vi "sub_qam_symbol_map_gen.vi"(9 "Gray code?":bool, 11 "M-QAM":i32) -> (3 "symbol map":cdb[](array[numeric]))   [LabVIEW 2014]
panel:
  out "Gray coded map":u32[][](array[numeric])
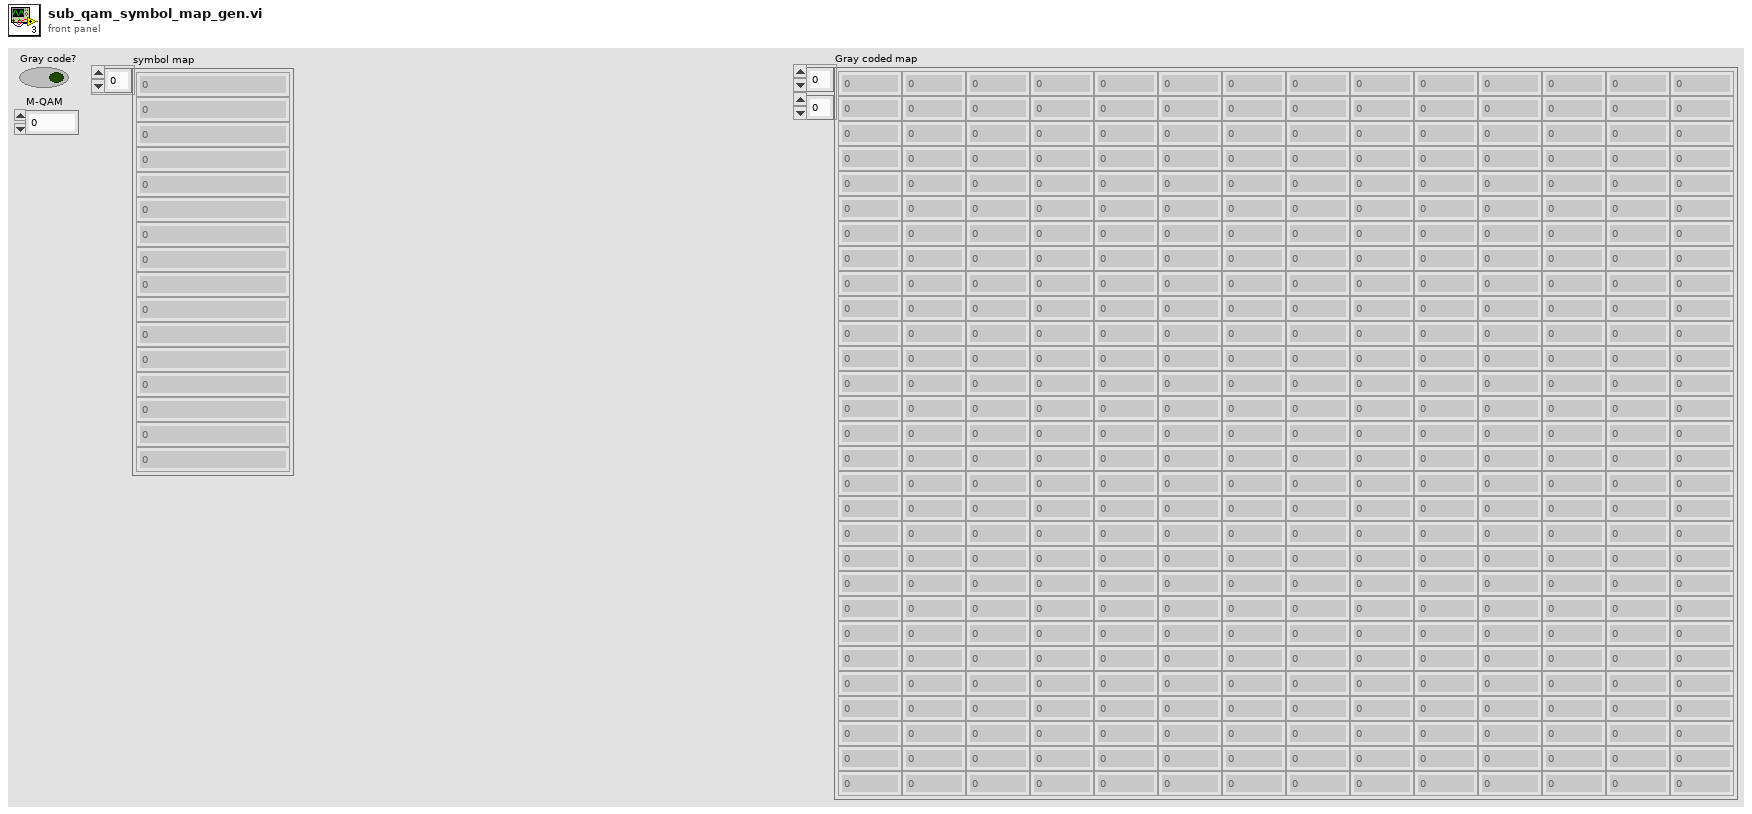
[diagram p1: front panel]
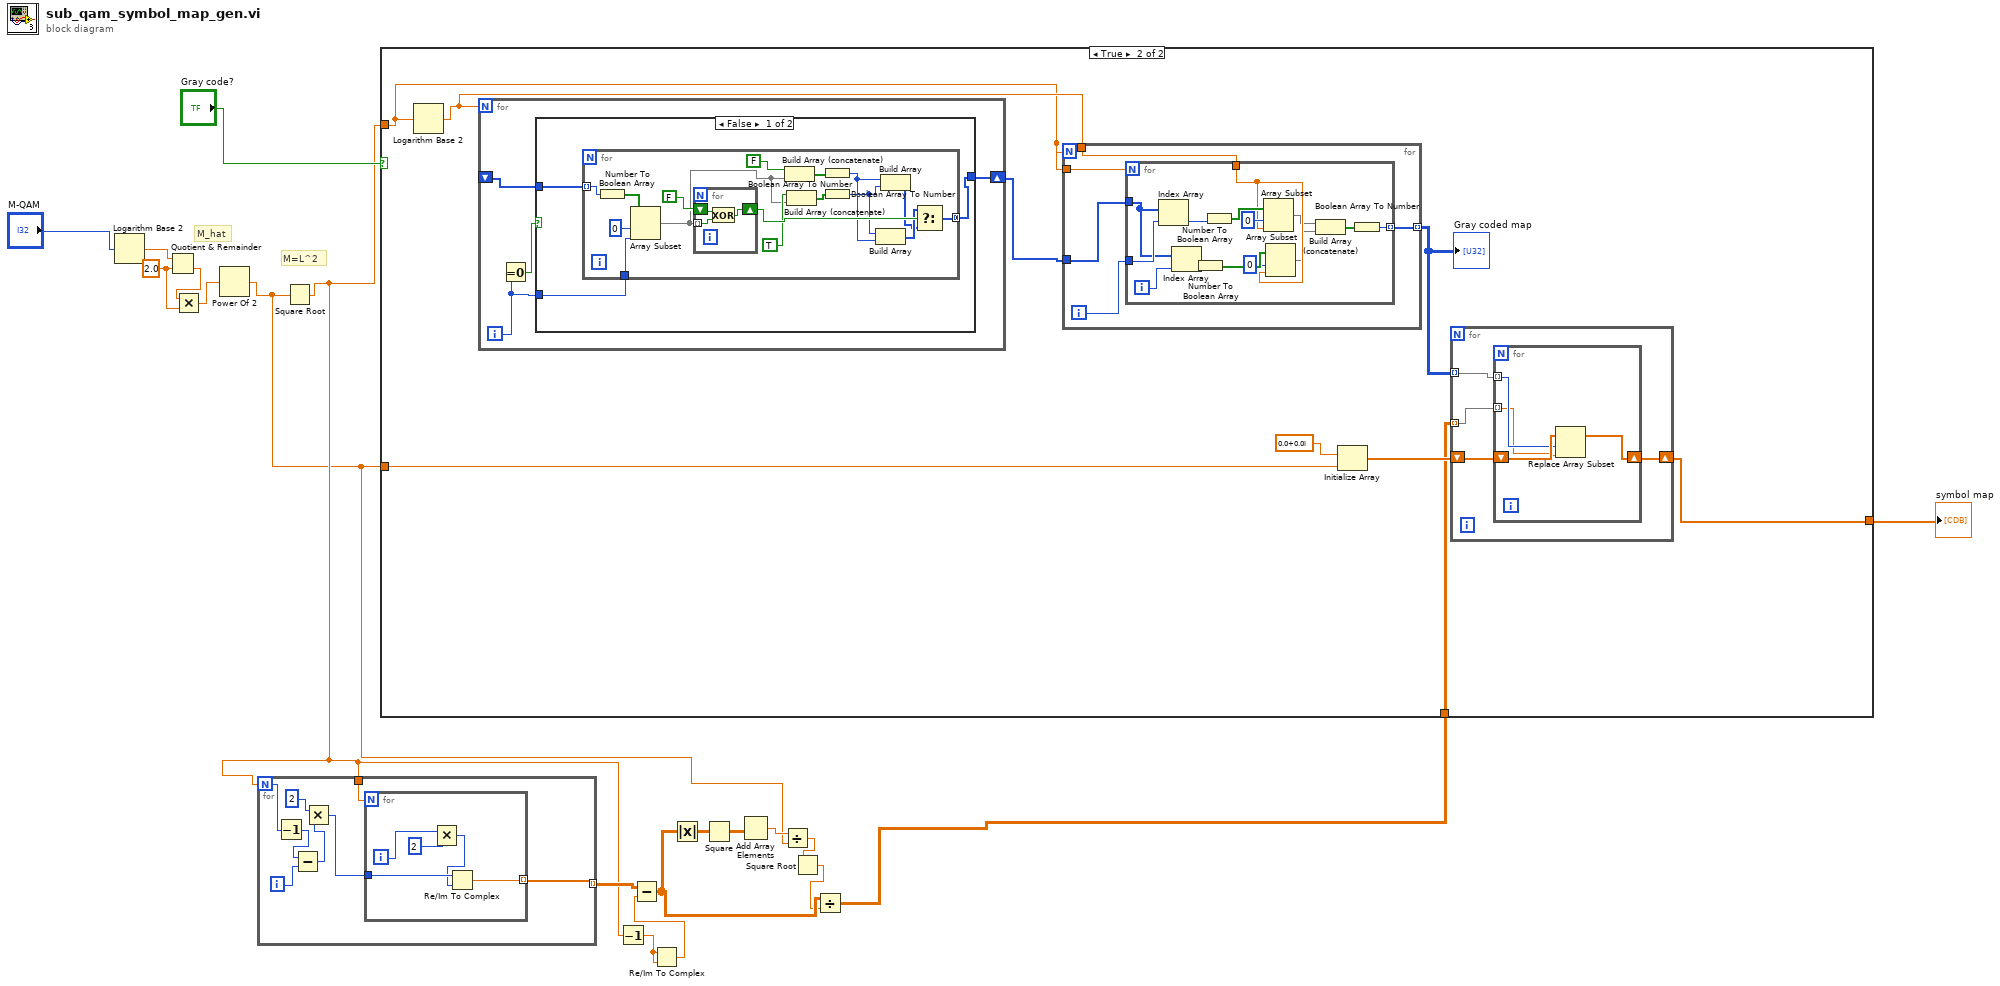
[diagram p0: block diagram]
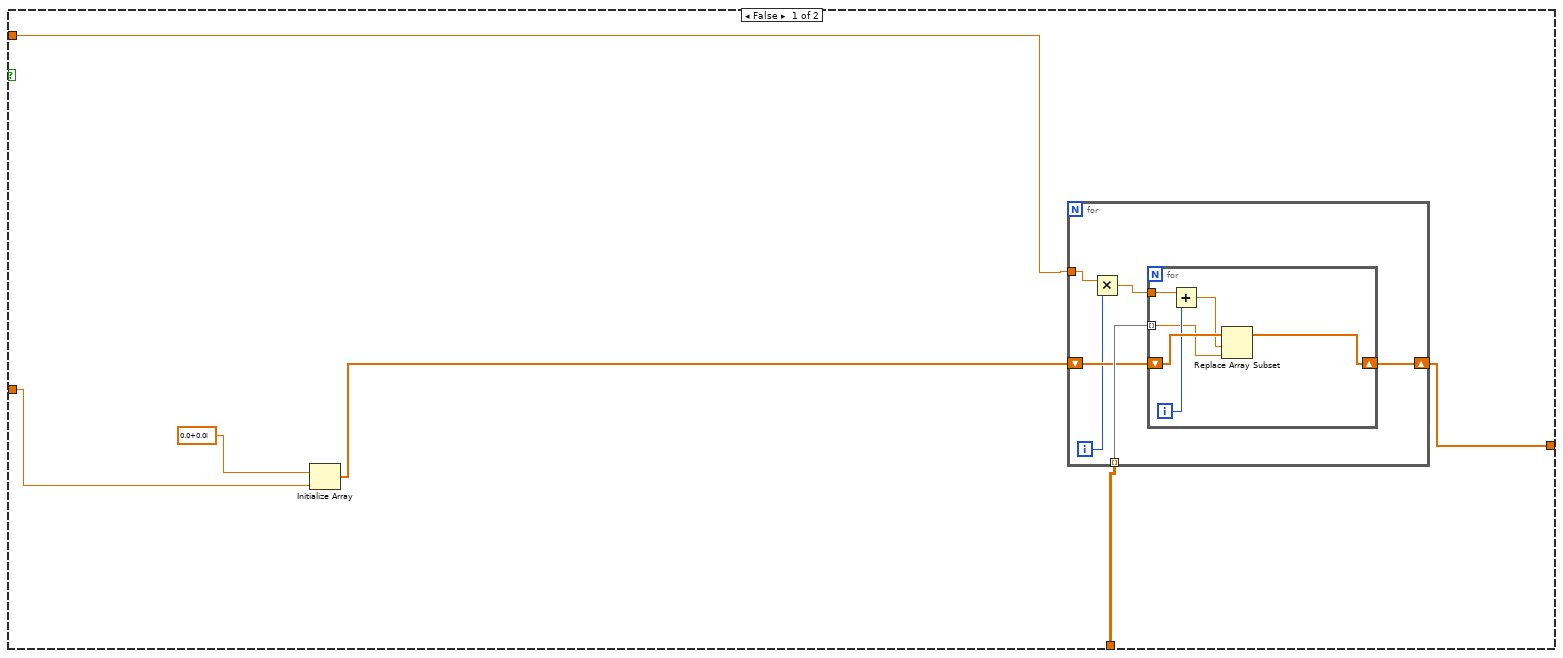
[diagram p2: hidden frame]
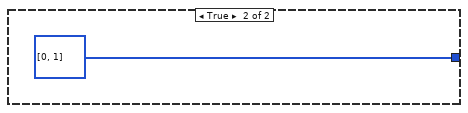
[diagram p3: hidden frame]
diagram:
  w15 = 2.0 ("y")
  # "M=L^2"
  # "M_hat"
  n1 = Logarithm Base 2(1:"M-QAM") -> (0:w18:dbl)
  n2 = Quotient & Remainder(x=w18, y=w15) -> (floor(x/y)=w16:dbl)  [unwired: 1 out]
  n3 = Multiply(x=w16, y=w15) -> (x*y=w14:dbl)
  n4 = Power Of 2(x=w14) -> (2^x=w1:dbl)
  n5 = Square Root(x=w1) -> (sqrt(x)=w3:dbl)
  n6 = for {
    N: w3 -> [w23]
    tunnel: w3 -> [w26]
    tunnel: [w24] -> w12 mode=indexing
    i -> [w21]
    n7 = Decrement(x=w23) -> (x-1=w22:i32)
    n8 = Subtract(x=w22, y=w21) -> (x-y=w20:i32)
    n9 = Multiply(x=2, y=w20) -> (x*y=w25:i32)
    n10 = for {
      N: w26 -> [_]
      tunnel: w25 -> [w29]
      tunnel: [w31] -> w24 mode=indexing
      i -> [w30]
      n11 = Multiply(x=w30, y=2) -> (x*y=w28:i32)
      n12 = Re/Im To Complex(1:w28, 2:w29) -> (0:w31:cdb)
    }
  }
  n13 = Decrement(x=w3) -> (x-1=w11:dbl)
  n14 = Re/Im To Complex(1:w11, 2:w11) -> (0:w10:cdb)
  n15 = Subtract(x=w12, y=w10) -> (x-y=w6:cdb[][])
  n16 = Absolute Value(x=w6) -> (abs(x)=w9:dbl[][])
  n17 = Square(x=w9) -> (x^2=w8:dbl[][])
  n18 = Add Array Elements(numeric array=w8) -> (sum=w7:dbl)
  n19 = Divide(x=w7, y=w1) -> (x/y=w5:dbl)
  n20 = Square Root(x=w5) -> (sqrt(x)=w4:dbl)
  n21 = Divide(x=w6, y=w4) -> (x/y=w2:cdb[][])
  n22 = case shown="True" "Gray code?" {
    tunnel: w3 -> [w34 w57]
    tunnel: [w33 w53] -> w13
    tunnel: w2 -> [w36 w52]
    tunnel: w1 -> [w37 w51]
    frame False {
      n23 = Initialize Array(cdb 0.0+0.0i, w37) -> (w35:cdb[])
      n24 = for {
        tunnel: w36 -> [w44] mode=indexing
        shift-right: [w39] -> w33
        shift-left: w35 -> [w43]
        tunnel: w34 -> [w42]
        i -> [w41]
        n25 = Multiply(x=w42, y=w41) -> (x*y=w40:dbl)
        n26 = for {
          tunnel: w44 -> [w46] mode=indexing
          shift-right: [w45] -> w39
          shift-left: w43 -> [w50]
          tunnel: w40 -> [w49]
          i -> [w48]
          n27 = Add(x=w49, y=w48) -> (x+y=w47:dbl)
          n28 = Replace Array Subset(array=w50, new element=w46, index=w47) -> (w45:cdb[])
        }
      }
    }
    frame True {
      n29 = Logarithm Base 2(1:w57) -> (0:w58:dbl)
      n30 = for {
        N: w58 -> [_]
        shift-right: [w89] -> w59
        shift-left: _ -> [w88]
        i -> [w87]
        n31 = Equal To 0?(x=w87) -> (x = 0?=w90:bool)
        n32 = case shown="False" w90 {
          tunnel: [w91 i32[] [0, 1]] -> w89
          tunnel: w88 -> [w93 _]
          tunnel: w87 -> [w92 _]
          frame False {
            n33 = for {
              tunnel: w93 -> [w109] mode=indexing
              tunnel: w92 -> [w106]
              tunnel: [w97] -> w91 mode=concatenating
              n34 = Number To Boolean Array(number=w109) -> (Boolean array=w108:bool[])
              n35 = Array Subset(array=w108, index=0, length=w106) -> (w94:bool[])
              n36 = for {
                shift-right: [w110] -> w104
                shift-left: FALSE -> [w112]
                tunnel: w94 -> [w111] mode=indexing
                n37 = Exclusive Or(1:w111, 2:w112) -> (0:w110:bool)
              }
              n38 = Build Array (concatenate)(FALSE, w94) -> (w103:bool[])
              n39 = Build Array (concatenate)(TRUE, w94) -> (w102:bool[])
              n40 = Boolean Array To Number(Boolean array=w103) -> (number=w100:u32)
              n41 = Boolean Array To Number(Boolean array=w102) -> (number=w101:u32)
              n42 = Build Array(w101, w100) -> (w99:u32[])
              n43 = Build Array(w100, w101) -> (w98:u32[])
              n44 = Select(t=w99, s=w104, f=w98) -> (s? t:f=w97:u32[])
            }
          }
          frame True {
          }
        }
      }
      n45 = for {
        N: w57 -> [_]
        tunnel: w59 -> [w72]
        tunnel: w58 -> [w70]
        tunnel: [w69] -> w56 mode=indexing
        tunnel: w57 -> [w68]
        i -> [w71]
        n46 = for {
          N: w68 -> [_]
          tunnel: w72 -> [w85]
          tunnel: w71 -> [w86]
          tunnel: w70 -> [w77]
          tunnel: [w73] -> w69 mode=indexing
          i -> [w84]
          n47 = Index Array(array=w85, index=w86) -> (element=w83:u32)
          n48 = Index Array(array=w85, index=w84) -> (element=w82:u32)
          n49 = Number To Boolean Array(number=w82) -> (Boolean array=w79:bool[])
          n50 = Number To Boolean Array(number=w83) -> (Boolean array=w81:bool[])
          n51 = Array Subset(array=w81, index=0, length=w77) -> (w76:bool[])
          n52 = Array Subset(array=w79, index=0, length=w77) -> (w75:bool[])
          n53 = Build Array (concatenate)(w76, w75) -> (w74:bool[])
          n54 = Boolean Array To Number(Boolean array=w74) -> (number=w73:u32)
        }
      }
      "Gray coded map" <- w56
      n55 = Initialize Array(cdb 0.0+0.0i, w51) -> (w54:cdb[])
      n56 = for {
        tunnel: w56 -> [w63] mode=indexing
        tunnel: w52 -> [w62] mode=indexing
        shift-right: [w60] -> w53
        shift-left: w54 -> [w61]
        n57 = for {
          tunnel: w63 -> [w66] mode=indexing
          tunnel: w62 -> [w65] mode=indexing
          shift-right: [w64] -> w60
          shift-left: w61 -> [w67]
          n58 = Replace Array Subset(array=w67, new element=w65, index=w66) -> (w64:cdb[])
        }
      }
    }
  }
  "symbol map" <- w13
